vi "Mass Compile Source.vi"(8 "Error In":errorcluster, 11 "Sync Source Config":T1) -> (0 "Error Out":errorcluster, 2 "Mass Compile Log":path, 3 "Sync Source Config":T1)   [LabVIEW 2011, in "LVH-Build-Tools.lvlib"]
uses:
  LVH-Build-Tools.lvlib
  Type Defs/Sync Source Configuration.ctl
  Type Defs/Installed Project.ctl
  Local Toolbox/_Installed LabVIEW Version.ctl
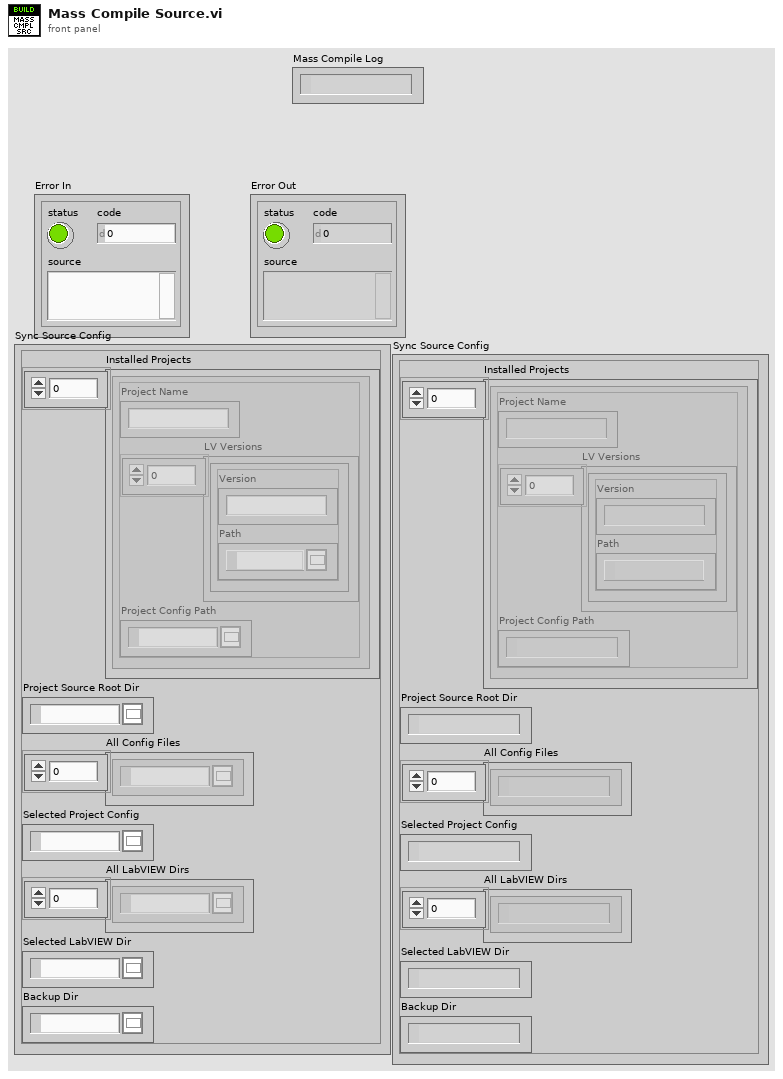
[diagram p1: front panel]
types:
  T1 = typedef "LVH-Build-Tools.lvlib/Sync Source Configuration.ctl" = cluster{"Installed Projects":T2[], "Project Source Root Dir":path, "All Config Files":path[], "Selected Project Config":path, "All LabVIEW Dirs":path[], "Selected LabVIEW Dir":path, "Backup Dir":path}
  T2 = typedef "LVH-Build-Tools.lvlib/Installed Project.ctl" = cluster{"Project Name":string, "LV Versions":T3[], "Project Config Path":path}
  T3 = typedef "LVH-Build-Tools.lvlib/_Installed LabVIEW Version.ctl" = cluster{"Version":string, "Path":path}
  T4 = enum32{"invalid app kind", "Development System", "Run Time System", "Student Edition", "Embedded LabVIEW", "Evaluation", "Custom"}
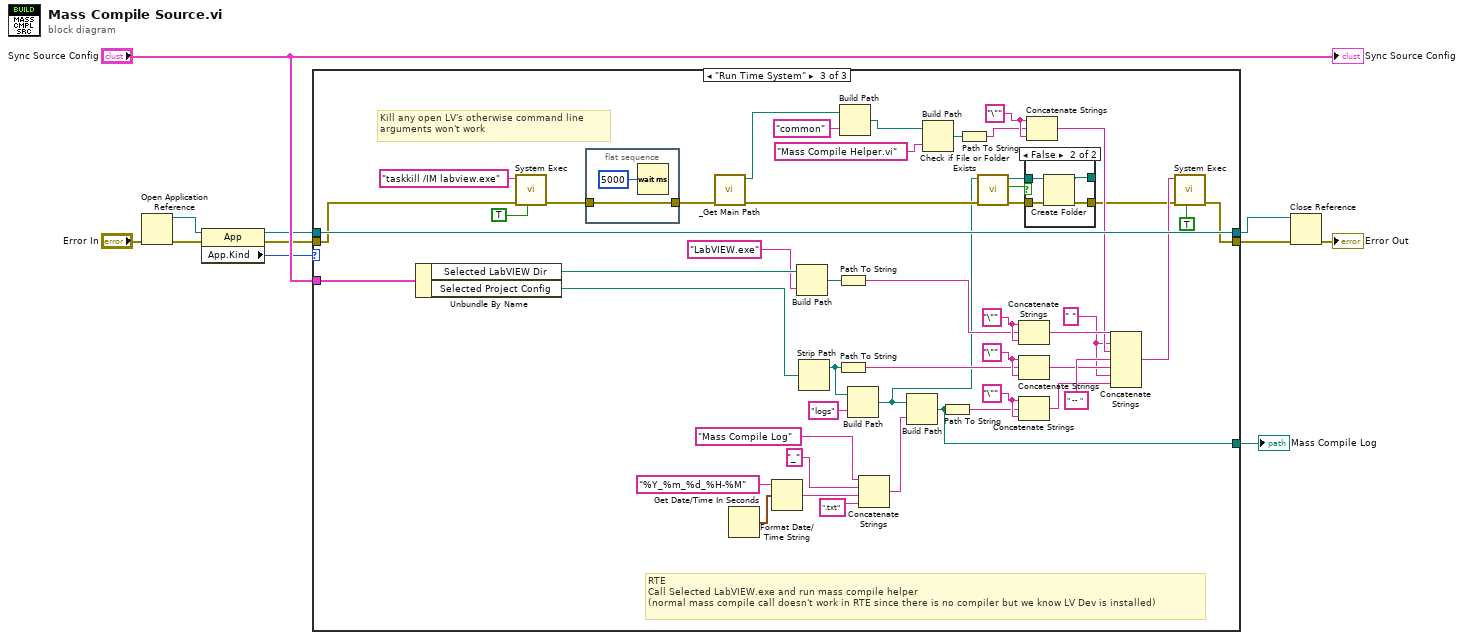
[diagram p0: block diagram]
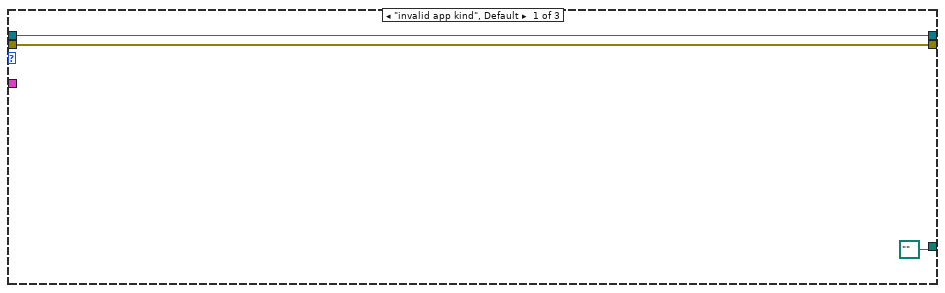
[diagram p2: hidden frame]
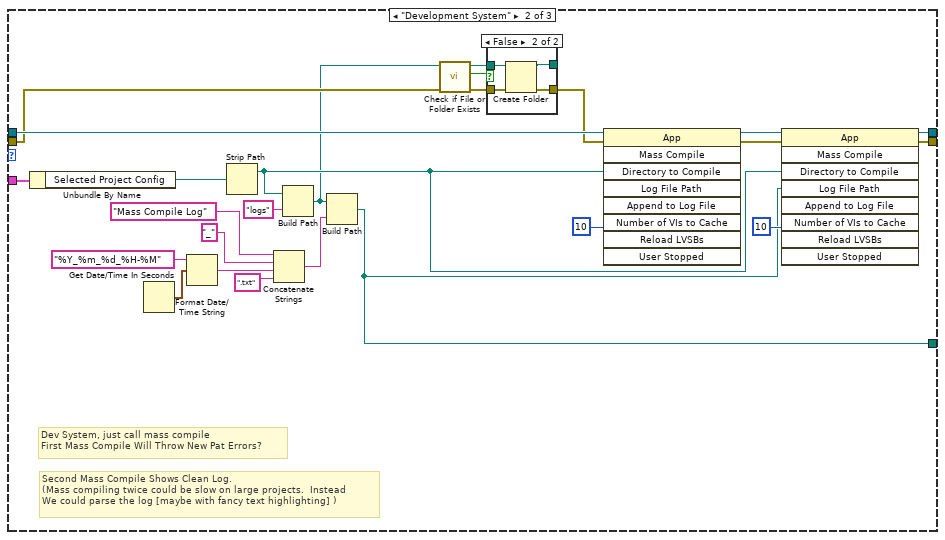
[diagram p3: hidden frame]
diagram:
  n1 = Open Application Reference(8:"Error In") -> (0:w6:errorcluster, 3:w5:refnum<vi>)  [unwired: 3 in]
  n2 = property class="App"(reference=w5, error in=w6) -> (reference out=w4:refnum<vi>, error out=w3:errorcluster, "App.Kind"=w2:T4)
  n3 = case shown="\"Run Time System\"" w2 {
    tunnel: [w13 w37 w67] -> w11
    tunnel: [w14 w36 w91] -> w10
    tunnel: "Sync Source Config" -> [_ w32 w94]
    tunnel: w4 -> [w14 w33 w91]
    tunnel: w3 -> [w13 w17 w58]
    tunnel: [path "" ("appended path") w16 w54] -> w1
    frame "invalid app kind", Default {
    }
    frame "Development System" {
      # "Second Mass Compile Shows Clean Log.\n(Mass compiling twice could be slow on large projects.  Instead \nWe could parse the log [maybe with fancy text highlighting] )"
      # "Dev System, just call mass compile\nFirst Mass Compile Will Throw New Pat Errors?"
      n4 = Unbundle By Name(w32) -> ("Selected Project Config"=w31:path)
      n5 = Get Date/Time In Seconds() -> (seconds since 1Jan1904=w30:timestamp)
      n6 = Format Date/Time String(time format string (%c)="%Y_%m_%d_%H-%M", seconds (now)=w30) -> (date/time string=w28:string)  [unwired: 1 in]
      n7 = Strip Path(path=w31) -> (stripped path=w24:path)  [unwired: 1 out]
      n8 = Concatenate Strings("Mass Compile Log" ("string"), "_" ("string"), w28, ".txt" ("string")) -> (w22:string)
      n9 = Build Path(base path=w24, name or relative path="logs") -> (appended path=w15:path)
      n10 = Build Path(base path=w15, name or relative path=w22) -> (appended path=w16:path)
      n11 = call <vilib>:"Check if File or Folder Exists.vi"("error in (no error)"=w17, "path"=w15) -> ("error out"=w19:errorcluster, "file or folder exists?"=w21:bool, "dup path"=w20:path)  [unwired: 7 in]
      n12 = case shown="False" w21 {
        tunnel: w20 -> [w40 w43]
        tunnel: [w41 w44] -> w18
        tunnel: w19 -> [w41 w45]
        tunnel: [w40 w42] -> _
        frame True {
        }
        frame False {
          n13 = Create Folder(path (use dialog)=w43, error in=w45) -> (created path=w42:path, error out=w44:errorcluster)  [unwired: 1 in, 1 out]
        }
      }
      n14 = invoke class="App" method="Mass Compile"(reference=w33, error in=w18, "Directory to Compile"=w24, "Number of VIs to Cache"=u32 10) -> (reference out=w38:refnum<vi>, error out=w39:errorcluster)  [unwired: 5 in, 7 out]
      n15 = invoke class="App" method="Mass Compile"(reference=w38, error in=w39, "Directory to Compile"=w24, "Log File Path"=w16, "Number of VIs to Cache"=u32 10) -> (reference out=w36:refnum<vi>, error out=w37:errorcluster)  [unwired: 4 in, 7 out]
    }
    frame "Run Time System" {
      w62 = "\"" ("string")
      w65 = "\"" ("string")
      w59 = " " ("string")
      w84 = "\"" ("string")
      w86 = "\"" ("string")
      # "Kill any open LV's otherwise command line \narguments won't work"
      # "RTE\nCall Selected LabVIEW.exe and run mass compile helper\n(normal mass compile call doesn't work in RTE since there is no compiler but we know LV Dev is installed)"
      n16 = Unbundle By Name(w94) -> ("Selected LabVIEW Dir"=w93:path, "Selected Project Config"=w77:path)
      n17 = call <vilib>:"System Exec.vi"("run minimized? (F)"=TRUE, "error in (no error)"=w58, "command line"="taskkill /IM labview.exe") -> ("error out"=w52:errorcluster)  [unwired: 5 in, 3 out]
      n18 = flat-sequence {
        tunnel: [w102] -> w53
        tunnel: w52 -> [w102]
        frame #0 {
          n19 = Wait (ms)(milliseconds to wait=u32 5000) -> ()  [unwired: 1 out]
        }
      }
      n20 = call "_Get Main Path.vi"("Error In"=w53) -> ("Error Out"=w48:errorcluster, "Main Dir"=w90:path)  [unwired: 8 in, 1 out]
      n21 = Get Date/Time In Seconds() -> (seconds since 1Jan1904=w74:timestamp)
      n22 = Format Date/Time String(time format string (%c)="%Y_%m_%d_%H-%M", seconds (now)=w74) -> (date/time string=w72:string)  [unwired: 1 in]
      n23 = Build Path(base path=w93, name or relative path="LabVIEW.exe") -> (appended path=w78:path)
      n24 = Strip Path(path=w77) -> (stripped path=w76:path)  [unwired: 1 out]
      n25 = Path To String(path=w78) -> (string=w85:string)
      n26 = Path To String(path=w76) -> (string=w63:string)
      n27 = Build Path(base path=w90, name or relative path="common") -> (appended path=w88:path)
      n28 = Build Path(base path=w76, name or relative path="logs") -> (appended path=w46:path)
      n29 = Concatenate Strings("Mass Compile Log" ("string"), "_" ("string"), w72, ".txt" ("string")) -> (w68:string)
      n30 = Build Path(base path=w46, name or relative path=w68) -> (appended path=w54:path)
      n31 = Build Path(base path=w88, name or relative path="Mass Compile Helper.vi") -> (appended path=w83:path)
      n32 = Path To String(path=w54) -> (string=w61:string)
      n33 = Path To String(path=w83) -> (string=w82:string)
      n34 = call <vilib>:"Check if File or Folder Exists.vi"("error in (no error)"=w48, "path"=w46) -> ("error out"=w49:errorcluster, "file or folder exists?"=w51:bool, "dup path"=w50:path)  [unwired: 7 in]
      n35 = Concatenate Strings(w86, w85, w86) -> (w81:string)
      n36 = Concatenate Strings(w65, w63, w65) -> (w64:string)
      n37 = Concatenate Strings(w62, w61, w62) -> (w60:string)
      n38 = case shown="False" w51 {
        tunnel: w50 -> [w95 w98]
        tunnel: [w96 w99] -> w47
        tunnel: w49 -> [w96 w100]
        tunnel: [w95 w97] -> _
        frame True {
        }
        frame False {
          n39 = Create Folder(path (use dialog)=w98, error in=w100) -> (created path=w97:path, error out=w99:errorcluster)  [unwired: 1 in, 1 out]
        }
      }
      n40 = Concatenate Strings(w84, w82, w84) -> (w80:string)
      n41 = Concatenate Strings(w81, w59, w80, " -- " ("string"), w64, w59, w60) -> (w66:string)
      n42 = call <vilib>:"System Exec.vi"("run minimized? (F)"=TRUE, "error in (no error)"=w47, "command line"=w66) -> ("error out"=w67:errorcluster)  [unwired: 5 in, 3 out]
    }
  }
  "Mass Compile Log" <- w1
  n43 = Close Reference(reference=w10, error in (no error)=w11) -> (error out=→"Error Out":errorcluster)
  "Sync Source Config" <- "Sync Source Config"
